vi "Extraction - MainUI.vi"() -> ()   [LabVIEW 2020]
uses:
  File Name Format.ctl
  <vilib>/addons/HF Network Analysis/Support VIs/Read SnP File (SnP).vi
  <vilib>/addons/HF Network Analysis/NI_HFNetworkAnalysis.lvlib
panel:
  in  "Tab Control":enum32{"Main", "Graphs", "Data Table"}(tab)
  in  "Device":T1
  in  "Copy comments":bool caption="Copy comments from \noriginal files (ISD de-embedding)"
  in  "SnP File Path":path
  in  "Filename has to include:":string="_DUT"
  in  "File name format":T2=enum."LV-framework, no file name"
  in  "Model":enum16{"pi", "tee"}(ring)
  in  "Freq for nominal \nvalues (MHz)":dbl=100.0
  in  "Ports":T3(ring)
  in  "Subtract stub":bool
  in  "Inductance (nH)":dbl=0.306
  in  "Capacitance (pF)":dbl=0.04
  out "Horizontal Progress Bar":u8(slide) scale=0.0..100.0
  in  "Play":bool
  in  "Exit":bool
  out "Status":string
  in  "Result File Path":path caption="Result File Path (empty: use the SnP-folder above)"
  in  "File extension":enum16{"Auto", "s1p", "s2p"}(ring)
  in  "Save extraction data":bool=TRUE
  in  "Save file index data":bool=TRUE
  in  "toJMP":bool caption="Save in JMP"
  out "Capa":cluster{"Frequencies (Hz) in":dbl[], dbl[]}[](graph) caption="Capacitance"
  out "R":cluster{"Frequencies (Hz) in":dbl[], dbl[]}(graph) caption="Resistance"
  out "Q":cluster{"Frequencies (Hz) in":dbl[], dbl[]}(graph)
  out "Error Out":errorcluster
  out "Heading":string[](array[string])
  out "Data":string[][](array[string])
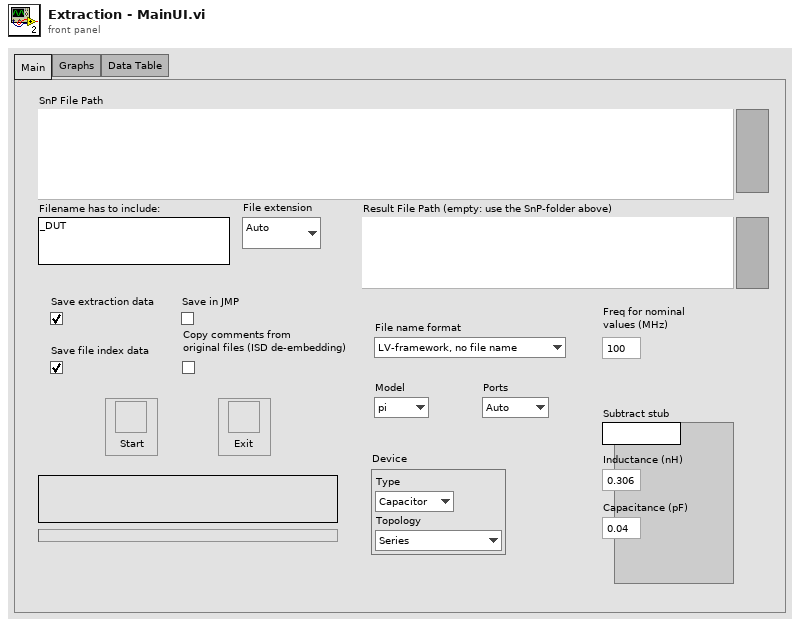
[diagram p1: front panel]
types:
  T1 = cluster{"Type":enum16{"Capacitor", "Switch"}, "Topology":enum16{"Series", "Parallel"}}
  T2 = typedef "File Name Format.ctl" = enum16{"none", "S-para, old", "S-para, new", "S-para, new, step", "ECP", "S-para, new+1", "WS1040", "S-para, new+5100", "S-para, new+5100, no step", "General, space limited", "General, underscore limited", "General, whitespace limited", "LV-framework", "LV-framework, no file name"}
  T3 = enum16{"Auto", "1-Port", "2-Port", "3-port", "4-port"}
  T4 = enum8{"Enabled", "Disabled", "Disabled and Grayed Out"}
  T5 = cluster{cluster{"Frequencies (Hz) in":dbl[], dbl[]}, cluster{"Frequencies (Hz) in":dbl[], dbl[]}, cluster{"Frequencies (Hz) in":dbl[], dbl[]}[]}
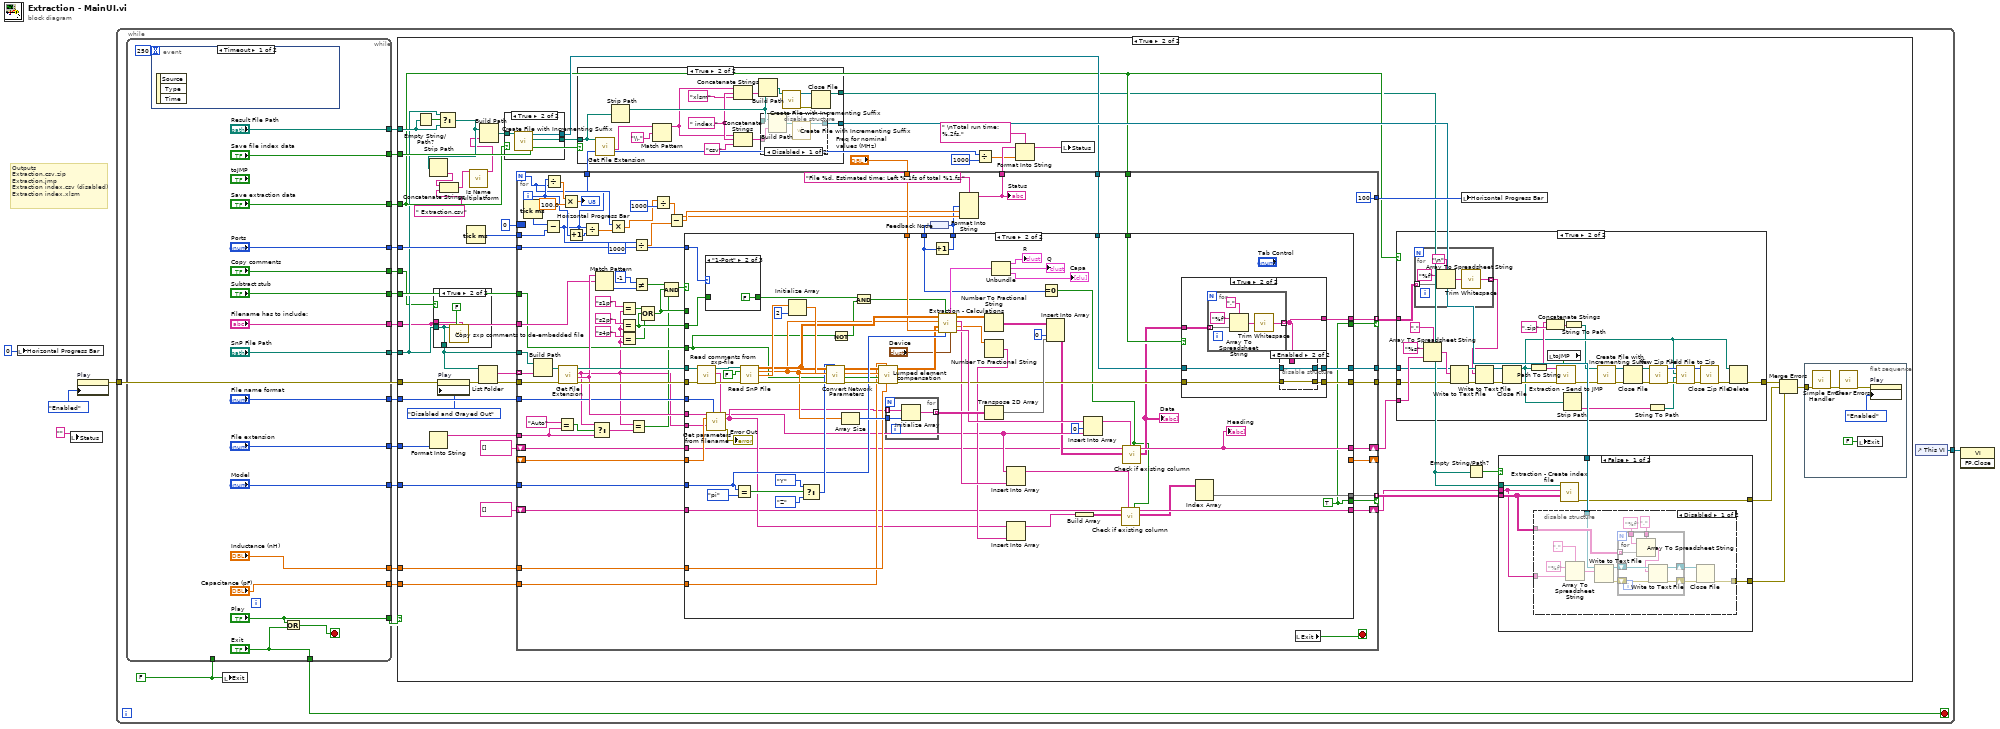
[diagram p0: block diagram]
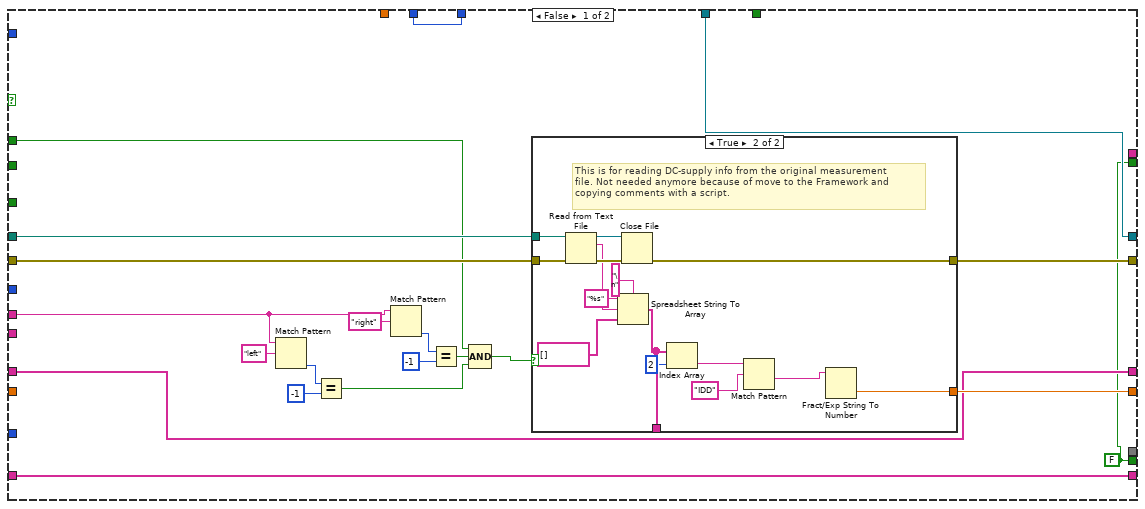
[diagram p10: hidden frame]
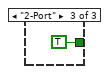
[diagram p13: hidden frame]
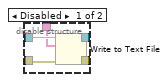
[diagram p15: hidden frame]
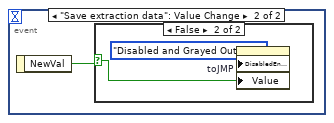
[diagram p16: hidden frame]
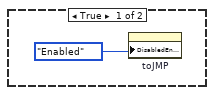
[diagram p17: hidden frame]
diagram:
  # "Outputs\nExtraction.csv.zip\nExtraction.jmp\nExtraction index.csv (disabled)\nExtraction index.xlsm"
  n1 = local write "Horizontal Progress Bar"(u8 0 ("Horizontal Progress Bar")) -> ()
  n2 = local write "Status"("" ("Status")) -> ()
  n3 = property on="Play" class="Bool"("DisabledEnum"=T4."Enabled" ("Disabled")) -> (error out=w3:errorcluster)  [unwired: 2 in, 1 out]
  n4 = while {
    tunnel: w3 -> [w12]
    tunnel: [w10] -> w1
    stop <- w13 stop-if-true
    w11 = FALSE ("Exit")
    n5 = while {
      tunnel: ["SnP File Path"] -> w23
      tunnel: ["Filename has to include:"] -> w22
      tunnel: ["Save extraction data"] -> w21
      tunnel: ["File name format"] -> w20
      tunnel: ["Model"] -> w19
      tunnel: ["Ports"] -> w18
      tunnel: ["Subtract stub"] -> w17
      tunnel: ["Inductance (nH)"] -> w16
      tunnel: ["Capacitance (pF)"] -> w15
      tunnel: ["Play"] -> w14
      tunnel: ["Exit"] -> w13
      tunnel: w11 -> [_]
      tunnel: ["File extension"] -> w9
      tunnel: ["Save file index data"] -> w8
      tunnel: ["Result File Path"] -> w7
      tunnel: ["Copy comments"] -> w6
      stop <- w386 stop-if-true
      n6 = event shown="[0] Timeout" {
        selector: _ -> [_ _]
        dyn-events: _ -> [_ _]
        timeout: 250 -> [_ _]
        event Timeout {
          n7 = event-data() -> ()  [unwired: 1 in, 3 out]
        }
        event "Save extraction data": Value Change {
          n8 = event-data() -> ("NewVal"=w396:bool)  [unwired: 1 in]
          n9 = case shown="False" w396 {
            selector: w396 -> [_ w398]
            frame True {
              n10 = property on="toJMP" class="Bool (strict)"("DisabledEnum"=T4."Enabled" ("Disabled")) -> ()  [unwired: 2 in, 2 out]
            }
            frame False {
              n11 = property on="toJMP" class="Bool (strict)"("DisabledEnum"=T4."Disabled and Grayed Out" ("Disabled"), "Value"=w398) -> ()  [unwired: 2 in, 2 out]
            }
          }
        }
      }
      n12 = Or(x="Play", y="Exit") -> (x .or. y?=w386:bool)
    }
    n13 = local write "Exit"(w11) -> ()
    n14 = case shown="True" w14 {
      tunnel: w23 -> [_ w27]
      tunnel: w22 -> [_ w24]
      tunnel: w21 -> [_ w43]
      tunnel: w20 -> [_ w72]
      tunnel: w19 -> [_ w71]
      tunnel: w18 -> [_ w69]
      tunnel: w17 -> [_ w68]
      tunnel: w16 -> [_ w67]
      tunnel: w15 -> [_ w66]
      tunnel: w12 -> [_ w62]
      tunnel: w9 -> [_ w53]
      tunnel: w8 -> [_ w45]
      tunnel: w7 -> [_ w44]
      tunnel: w6 -> [_ w26]
      frame False {
      }
      frame True {
        n15 = Empty String/Path?(string/path=w44) -> (empty?=w54:bool)
        n16 = Format Into String(w53) -> (resulting string=w52:string)  [unwired: 3 in, 1 out]
        n17 = case shown="True" w26 {
          tunnel: w27 -> [w78 w80]
          tunnel: [w78 w80] -> w25
          tunnel: w24 -> [_ w79]
          frame False {
          }
          frame True {
            n18 = call "Copy sxp comments to de-embedded file.vi"("Filename has to include:"=w79, "Standalone"=FALSE, "SnP File Path"=w80) -> ()  [unwired: 9 in]
          }
        }
        n19 = property on="Play" class="Bool"(error in=w62, "DisabledEnum"=T4."Disabled and Grayed Out" ("Disabled")) -> (error out=w63:errorcluster)  [unwired: 1 in, 1 out]
        n20 = Select(t=w27, s=w54, f=w44) -> (s? t:f=w36:path)
        n21 = Strip Path(path=w36) -> (name=w35:string)  [unwired: 1 out]
        n22 = Concatenate Strings(w35, " Extraction.csv" ("string")) -> (w34:string)
        n23 = Tick Count (ms)() -> (millisecond timer value=w61:u32)
        n24 = call <vilib>:"Is Name Multiplatform.vi"("filename"=w34) -> ("suggested filename"=w32:string)  [unwired: 6 in, 4 out]
        n25 = List Folder(path=w25, error in=w63) -> (filenames=w77:string[], error out=w76:errorcluster)  [unwired: 2 in, 2 out]
        n26 = Build Path(base path=w36, name or relative path=w32) -> (appended path=w75:path)
        n27 = case shown="True" w43 {
          tunnel: w75 -> [w147 w150]
          tunnel: [w147 w149] -> w47
          tunnel: [_ w148] -> w46
          frame False {
          }
          frame True {
            n28 = call <vilib>:"Create File with Incrementing Suffix.vi"("file path"=w150) -> ("actual path"=w149:path, "refnum out"=w148:refnum<file>)  [unwired: 8 in, 1 out]
          }
        }
        n29 = for {
          N -> [w202]
          tunnel: w25 -> [w232]
          tunnel: [w242] -> w73
          tunnel: w76 -> [w237]
          tunnel: w77 -> [w235] mode=indexing
          tunnel: w24 -> [w229]
          shift-right: [w228] -> _
          shift-left: _ -> [w227]
          tunnel: w43 -> [w226]
          tunnel: w46 -> [w225]
          tunnel: [w224] -> w74
          tunnel: w72 -> [w223]
          tunnel: w71 -> [w220]
          tunnel: "Freq for nominal \nvalues (MHz)" -> [w219]
          tunnel: w69 -> [w217]
          tunnel: w68 -> [w216]
          tunnel: w67 -> [w215]
          tunnel: w66 -> [w214]
          tunnel: [u8 100 ("Horizontal Progress Bar")] -> w65
          tunnel: w61 -> [w207]
          tunnel: [w194] -> w59
          tunnel: [w193] -> w58
          tunnel: w52 -> [w190]
          tunnel: [w187] -> w51 mode=indexing if=w186
          border: 0 -> [_]
          shift-right: [w182] -> w31
          shift-left: string[] [] ("Main Heading") -> [w181]
          shift-right: [w185] -> w50
          shift-left: string[] [] ("Main Heading") -> [w180]
          tunnel: [w179] -> w28 mode=indexing if=w178
          i -> [w205]
          stop <- w209 stop-if-true
          n30 = Tick Count (ms)() -> (millisecond timer value=w206:u32)
          n31 = Build Path(base path=w232, name or relative path=w235) -> (appended path=w234:path)
          n32 = Subtract(x=w206, y=w207) -> (x-y=w194:u32)
          n33 = Divide(x=w205, y=w202) -> (x/y=w213:dbl)
          n34 = Equal?(x="Auto" ("y"), y=w190) -> (x = y?=w191:bool)
          n35 = call <vilib>:"Get File Extension.vi"("error in (no error)"=w237, "file"=w234) -> ("error out"=w236:errorcluster, "filename without extension"=w230:string, "lowercase file extension"=w176:string, "dup file"=w231:path)  [unwired: 5 in, 1 out]
          n36 = Multiply(x=w213, y=100.0) -> (x*y=→"Horizontal Progress Bar":dbl)
          n37 = Increment(x=w205) -> (x+1=w204:i32)
          n38 = Divide(x=w194, y=w204) -> (x/y=w203:dbl)
          n39 = Select(t=w176, s=w191, f=w190) -> (s? t:f=w189:string)
          n40 = Match Pattern(string=w230, regular expression=w229) -> (offset past match=w233:i32)  [unwired: 1 in, 3 out]
          n41 = Multiply(x=w202, y=w203) -> (x*y=w196:dbl)
          n42 = Equal?(x="s1p" ("regular expression"), y=w176) -> (x = y?=w221:bool)
          n43 = Equal?(x="s2p" ("regular expression"), y=w176) -> (x = y?=w218:bool)
          n44 = Equal?(x="s4p" ("regular expression"), y=w176) -> (x = y?=w175:bool)
          n45 = Equal?(x=w176, y=w189) -> (x = y?=w188:bool)
          n46 = Divide(x=w194, y=u32 1000) -> (x/y=w199:dbl)
          n47 = Not Equal?(x=-1, y=w233) -> (x != y?=w241:bool)
          n48 = Compound Arithmetic op=OR(w221, w218, w175) -> (w208:bool)
          n49 = Divide(x=w196, y=u32 1000) -> (x/y=w195:dbl)
          n50 = Compound Arithmetic op=AND(w241, w208, w188) -> (w238:bool)
          n51 = Subtract(x=w195, y=w199) -> (x-y=w198:dbl)
          n52 = feedback #1() -> (w184:i32)
          n53 = case shown="True" w238 {
            tunnel: w231 -> [w260 w311]
            tunnel: [w259 w338] -> w242
            tunnel: w236 -> [w261 w312]
            tunnel: w230 -> [w262 w345]
            tunnel: [w258 _] -> w228
            tunnel: w227 -> [_ w339]
            tunnel: w226 -> [_ w337]
            tunnel: w225 -> [w257 w335]
            tunnel: [w257 w334] -> w224
            tunnel: w223 -> [_ w333]
            tunnel: w218 -> [_ w324]
            tunnel: w220 -> [_ w327]
            tunnel: w219 -> [_ w326]
            tunnel: w217 -> [_ w325]
            tunnel: w176 -> [_ w323]
            tunnel: w216 -> [_ w317]
            tunnel: w215 -> [_ w315]
            tunnel: w214 -> [_ w314]
            tunnel: w208 -> [w247 _]
            tunnel: [w244 w291] -> w185
            tunnel: [w243 w283] -> w186
            tunnel: [_ w285] -> w187
            tunnel: w184 -> [w246 w282]
            tunnel: [w246 w307] -> w183
            tunnel: [w245 w296] -> w182
            tunnel: w181 -> [w245 w281]
            tunnel: w180 -> [w244 w289]
            tunnel: [_ w284] -> w179
            tunnel: [w243 w283] -> w178
            frame False {
              w243 = FALSE
              n54 = Match Pattern(string=w262, regular expression="left") -> (offset past match=w254:i32)  [unwired: 1 in, 3 out]
              n55 = Equal?(x=w254, y=-1) -> (x = y?=w249:bool)
              n56 = Match Pattern(string=w262, regular expression="right") -> (offset past match=w251:i32)  [unwired: 1 in, 3 out]
              n57 = Equal?(x=w251, y=-1) -> (x = y?=w250:bool)
              n58 = Compound Arithmetic op=AND(w247, w250, w249) -> (w248:bool)
              n59 = case shown="True" w248 {
                tunnel: w261 -> [w263 w276]
                tunnel: w260 -> [_ w275]
                tunnel: [w263 w274] -> w259
                tunnel: [_ w269] -> _
                tunnel: [_ w264] -> w258
                frame False {
                }
                frame True {
                  # "This is for reading DC-supply info from the original measurement \nfile. Not needed anymore because of move to the Framework and \ncopying comments with a script."
                  n60 = Read from Text File(file (use dialog)=w275, error in=w276) -> (refnum out=w277:refnum<file>, text=w273:string, error out=w278:errorcluster)  [unwired: 2 in, 1 out]
                  n61 = Spreadsheet String To Array(delimiter (Tab)="\n" ("format string"), format string="%s", spreadsheet string=w273, array type (2D Dbl)=string[] []) -> (array=w269:string[])
                  n62 = Close File(refnum=w277, error in=w278) -> (error out=w274:errorcluster)  [unwired: 1 out]
                  n63 = Index Array(array=w269, index=2) -> (element=w266:string)
                  n64 = Match Pattern(string=w266, regular expression="IDD" ("format string")) -> (after substring=w265:string)  [unwired: 1 in, 3 out]
                  n65 = Fract/Exp String To Number(string=w265) -> (number=w264:dbl)  [unwired: 3 in, 1 out]
                }
              }
            }
            frame True {
              w283 = TRUE
              n66 = call "Read comments from sxp-file.vi"("error in (no error)"=w312, "file path"=w311) -> ("error out"=w309:errorcluster, "Comment lines"=w308:string[], "file path out"=w310:path)  [unwired: 7 in]
              n67 = case shown="\"1-Port\"" w325 {
                tunnel: w324 -> [w353 _ _]
                tunnel: [w353 FALSE TRUE] -> w319
                frame "Auto", Default {
                }
                frame "1-Port" {
                }
                frame "2-Port" {
                }
              }
              n68 = call "Get parameters from filename.vi"("Filename"=w345, "File name format"=w333, "Comment lines"=w308, "Idd"=w339, "extension"=w323) -> ("Heading"=w297:string[], "Info"=w298:string[], "Error Out"=→"Error Out":errorcluster)  [unwired: 6 in, 2 out]
              n69 = Equal?(x=w327, y=enum16{"pi", "tee"}."pi") -> (x = y?=w328:bool)
              n70 = call-poly <vilib>:"Read SnP File.vi"("SnP File Path"=w310, "Swap Ports (False)"=FALSE, "Error In"=w309) -> ("S-parameters"=w346:cdb[][], "Frequencies (Hz)"=w322:dbl[], "Z0 (Ohm)"=w350:cdb, "Error Out"=w351:errorcluster)  [unwired: 9 in]
              n71 = Initialize Array(w350, 2 ("dimension size")) -> (w348:cdb[])
              n72 = Select(t=enum16{"Y", "Z"}."Y" ("Parameters to convert"), s=w328, f=enum16{"Y", "Z"}."Z" ("Parameters to convert")) -> (s? t:f=w330:enum16{"Y", "Z"})
              n73 = call "Convert Network Parameters.vi"("Parameters to convert"=w330, "error in (no error)"=w351, "Zc (Ohm)"=w348, "S-par Array In"=w346) -> ("error out"=w336:errorcluster, "Y/Z Array Out"=w320:cdb[][])  [unwired: 5 in, 1 out]
              n74 = Not(x=w317) -> (.not. x?=w316:bool)
              n75 = Array Size(array=w322) -> (size(s)=w344:i32)
              n76 = And(x=w319, y=w316) -> (x .and. y?=w318:bool)
              n77 = call "Lumped element compensation.vi"("Inductance (nH)"=w315, "Capacitance (pF)"=w314, "Subtract stub"=w317, "Frequencies (Hz)"=w322, "Y/Z Array Out in"=w320) -> ("Y/Z Array Out out"=w321:cdb[][])  [unwired: 6 in]
              n78 = for {
                tunnel: w298 -> [w378] mode=indexing
                tunnel: w344 -> [w377]
                tunnel: [w376] -> w342 mode=indexing
                n79 = Initialize Array(w378, w377) -> (w376:string[])
              }
              n80 = Increment(x=w282) -> (x+1=w307:i32)
              n81 = call "Extraction - Calculations.vi"("Device"="Device", "Model"=w327, "2-port?"=w318, "Freq for nominal C (MHz)"=w326, "Y/Z-parameters"=w321, "Frequencies (Hz) in"=w322, "S-parameters"=w346) -> ("Heading"=w340:string[], "index file values"=w300:dbl[], "index file heading"=w301:string[], "Frequency,C, R, Q/-IL, L, Cshunt1/2, Rshunt1/2, Lshunt1/2, SRF"=w306:dbl[][], "Graphs"=w305:T5)
              n82 = Number To Fractional String(number=w306) -> (F-format string=w347:string[][])  [unwired: 3 in]
              n83 = Number To Fractional String(number=w300) -> (F-format string=w299:string[])  [unwired: 3 in]
              n84 = Transpose 2D Array(2D array=w342) -> (transposed array=w343:string[][])
              n85 = Unbundle(w305) -> (→"R":cluster{"Frequencies (Hz) in":dbl[], dbl[]}, →"Q":cluster{"Frequencies (Hz) in":dbl[], dbl[]}, →"Capa":cluster{"Frequencies (Hz) in":dbl[], dbl[]}[])
              n86 = Insert Into Array(array=w297, new element=w301) -> (w290:string[])  [unwired: 1 in]
              n87 = Insert Into Array(array=w298, new element=w299) -> (w288:string[])  [unwired: 1 in]
              n88 = Equal To 0?(x=w282) -> (x = 0?=w280:bool)
              n89 = Insert Into Array(array=w347, index (col)=0 ("disabled index (col)"), new element=w343) -> (w293:string[][])  [unwired: 1 in]
              n90 = Build Array(w288) -> (w287:string[][])
              n91 = Insert Into Array(array=w340, index=0, new element=w297) -> (w294:string[])
              n92 = call "Check if existing column.vi"("Init"=w280, "New Heading"=w290, "New Data"=w287, "Main Heading in"=w289) -> ("New Data out"=w286:string[][], "Main Heading"=w291:string[])  [unwired: 6 in]
              n93 = call "Check if existing column.vi"("Init"=w280, "New Heading"=w294, "New Data"=w293, "Main Heading in"=w281) -> ("New Data out"=w292:string[][], "Main Heading"=w296:string[])  [unwired: 6 in]
              "Data" <- w292
              "Heading" <- w296
              n94 = case shown="True" w337 {
                tunnel: [w357 w360] -> w338
                tunnel: w292 -> [_ w363]
                tunnel: w336 -> [w357 w362]
                tunnel: w335 -> [w356 w361]
                tunnel: [w356 w359] -> w334
                tunnel: [_ w358] -> w284
                frame False {
                }
                frame True {
                  n95 = for {
                    tunnel: w363 -> [w373] mode=indexing
                    tunnel: [w371] -> w358 mode=indexing
                    n96 = Array To Spreadsheet String(delimiter (Tab)=",", array=w373, 3:"%f" ("format string")) -> (spreadsheet string=w372:string)
                    n97 = call <vilib>:"Trim Whitespace.vi"("string"=w372) -> ("trimmed string"=w371:string)  [unwired: 1 in]
                  }
                  n98 = disable-structure shown="Enabled" {
                    disable-tunnel: w362 -> [w368 w369]
                    disable-tunnel: w361 -> [w367 w370]
                    disable-tunnel: [w366 w369] -> w360
                    disable-tunnel: [w365 w370] -> w359
                    disable-tunnel: w358 -> [w364 _]
                    frame Disabled {
                      n99 = Write to Text File(file (use dialog)=w367, text=w364, error in=w368) -> (refnum out=w365:refnum<file>, error out=w366:errorcluster)  [unwired: 1 in, 1 out]
                    }
                    frame Enabled {
                    }
                  }
                }
              }
              n100 = Index Array(array=w286) -> (element=w285:string[])  [unwired: 2 in]
            }
          }
          n101 = feedback-in #1(w183) -> ()
          n102 = Format Into String(format string="File %d. Estimated time: Left %.1fs of total %1.fs.", w183, w198, w195) -> (resulting string=w193:string)  [unwired: 2 in, 1 out]
          "Status" <- w193
          n103 = local read "Exit"() -> (w209:bool)
        }
        n104 = case shown="True" w45 {
          tunnel: [_ w169] -> w49
          tunnel: [_ w161] -> w38
          tunnel: w47 -> [_ w160]
          frame False {
          }
          frame True {
            w165 = " index." ("string")
            n105 = call <vilib>:"Get File Extension.vi"("file"=w160) -> ("filename without extension"=w158:string)  [unwired: 6 in, 4 out]
            n106 = Strip Path(path=w160) -> (stripped path=w166:path)  [unwired: 1 out]
            n107 = Match Pattern(string=w158, regular expression="\\.") -> (before substring=w157:string)  [unwired: 1 in, 3 out]
            n108 = Concatenate Strings(w157, w165, "xlsm" ("string")) -> (w167:string)
            n109 = Concatenate Strings(w157, w165, "csv" ("string")) -> (w170:string)
            n110 = Build Path(base path=w166, name or relative path=w167) -> (appended path=w168:path)
            n111 = disable-structure shown="Disabled" {
              disable-tunnel: w170 -> [w173 _]
              disable-tunnel: [w172 _] -> w169
              disable-tunnel: w166 -> [w171 _]
              frame Disabled {
                n112 = Build Path(base path=w171, name or relative path=w173) -> (appended path=w174:path)
                n113 = call <vilib>:"Create File with Incrementing Suffix.vi"("file path"=w174) -> ("refnum out"=w172:refnum<file>)  [unwired: 8 in, 2 out]
              }
              frame Enabled {
              }
            }
            n114 = call <vilib>:"Create File with Incrementing Suffix.vi"("file path"=w168) -> ("error out"=w162:errorcluster, "refnum out"=w163:refnum<file>)  [unwired: 8 in, 1 out]
            n115 = Close File(refnum=w163, error in=w162) -> (path=w161:path)  [unwired: 1 out]
          }
        }
        n116 = Divide(x=w59, y=u32 1000) -> (x/y=w55:dbl)
        n117 = Format Into String(format string=" \nTotal run time: %.2fs.", initial string=w58, w55) -> (resulting string=w57:string)  [unwired: 1 in, 1 out]
        n118 = local write "Status"(w57) -> ()
        n119 = case shown="True" w43 {
          tunnel: w74 -> [_ w135]
          tunnel: w73 -> [w109 w134]
          tunnel: [w109 w117] -> w40
          tunnel: w31 -> [_ w137]
          tunnel: w28 -> [_ w129]
          frame False {
          }
          frame True {
            n120 = for {
              tunnel: w129 -> [w144] mode=indexing
              tunnel: [w142] -> w128 mode=indexing
              n121 = Array To Spreadsheet String(delimiter (Tab)="\n", array=w144, 3:"%f" ("format string")) -> (spreadsheet string=w143:string)
              n122 = call <vilib>:"Trim Whitespace.vi"("string"=w143) -> ("trimmed string"=w142:string)  [unwired: 1 in]
            }
            n123 = Array To Spreadsheet String(delimiter (Tab)=",", array=w137, 3:"%s" ("format string")) -> (spreadsheet string=w136:string)
            n124 = Write to Text File(file (use dialog)=w135, text=w136, error in=w134) -> (refnum out=w133:refnum<file>, error out=w132:errorcluster)  [unwired: 1 in, 1 out]
            n125 = Write to Text File(file (use dialog)=w133, text=w128, error in=w132) -> (refnum out=w131:refnum<file>, error out=w130:errorcluster)  [unwired: 1 in, 1 out]
            n126 = Close File(refnum=w131, error in=w130) -> (path=w116:path, error out=w140:errorcluster)
            n127 = Path To String(path=w116) -> (string=w119:string)
            n128 = Concatenate Strings(w119, ".zip" ("name or relative path")) -> (w126:string)
            n129 = local read "toJMP"() -> (w141:bool)
            n130 = call "Extraction - Send to JMP.vi"("Send to JMP"=w141, "Error In"=w140, "filename"=w119) -> ("Error Out"=w111:errorcluster)  [unwired: 8 in]
            n131 = Strip Path(path=w116) -> (name=w121:string)  [unwired: 1 out]
            n132 = String To Path(string=w126) -> (path=w113:path)
            n133 = call <vilib>:"Create File with Incrementing Suffix.vi"("error in (no error)"=w111, "file path"=w113) -> ("error out"=w114:errorcluster, "refnum out"=w115:refnum<file>)  [unwired: 7 in, 1 out]
            n134 = Close File(refnum=w115, error in=w114) -> (path=w112:path, error out=w110:errorcluster)
            n135 = String To Path(string=w121) -> (path=w120:path)
            n136 = call <vilib>:"New Zip File.vi"("error in (no error)"=w110, "target"=w112) -> ("error out"=w125:errorcluster, "zip file out"=w124:i64)  [unwired: 3 in, 1 out]
            n137 = call <vilib>:"Add File to Zip.vi"("error in (no error)"=w125, "destination path in zip"=w120, "source file path"=w116, "zip file in"=w124) -> ("error out"=w122:errorcluster, "zip file out"=w123:i64)  [unwired: 6 in]
            n138 = call <vilib>:"Close Zip File.vi"("error in (no error)"=w122, "zip file in"=w123) -> ("error out"=w118:errorcluster)  [unwired: 5 in]
            n139 = Delete(path (use dialog)=w116, error in=w118) -> (error out=w117:errorcluster)  [unwired: 3 in, 2 out]
          }
        }
        n140 = local write "Horizontal Progress Bar"(w65) -> ()
        n141 = Empty String/Path?(string/path=w38) -> (empty?=w37:bool)
        n142 = case shown="False" w37 {
          tunnel: w51 -> [w87 _]
          tunnel: w38 -> [w86 _]
          tunnel: w50 -> [w85 _]
          tunnel: w49 -> [w84 _]
          tunnel: [w83 _] -> w42
          tunnel: [w82 _] -> w41
          frame False {
            n143 = disable-structure shown="Disabled" {
              disable-tunnel: w87 -> [w100 _]
              disable-tunnel: w85 -> [w99 _]
              disable-tunnel: w84 -> [w98 _]
              disable-tunnel: [w88 _] -> w83
              frame Disabled {
                n144 = Array To Spreadsheet String(delimiter (Tab)=",", array=w99, 3:"%f" ("format string")) -> (spreadsheet string=w91:string)
                n145 = Write to Text File(file (use dialog)=w98, text=w91) -> (refnum out=w96:refnum<file>, error out=w97:errorcluster)  [unwired: 2 in, 1 out]
                n146 = for {
                  tunnel: w100 -> [w102] mode=indexing
                  shift-right: [w106] -> w95
                  shift-left: w96 -> [w107]
                  shift-right: [w105] -> w94
                  shift-left: w97 -> [w108]
                  tunnel: "," ("delimiter (Tab)") -> [w104]
                  tunnel: "%f" ("format string") -> [w103]
                  n147 = Array To Spreadsheet String(delimiter (Tab)=w104, array=w102, 3:w103) -> (spreadsheet string=w101:string)
                  n148 = Write to Text File(file (use dialog)=w107, text=w101, error in=w108) -> (refnum out=w106:refnum<file>, error out=w105:errorcluster)  [unwired: 1 in, 1 out]
                }
                n149 = Close File(refnum=w95, error in=w94) -> (error out=w88:errorcluster)  [unwired: 1 out]
              }
              frame Enabled {
              }
            }
            n150 = call "Extraction - Create index file.vi"("Data"=w87, "Heading"=w85, "report file path"=w86) -> ("Error Out"=w82:errorcluster)  [unwired: 8 in]
          }
          frame True {
          }
        }
        n151 = Merge Errors(w40, w41, w42) -> (w39:errorcluster)
        n152 = flat-sequence {
          tunnel: w39 -> [w152]
          frame #0 {
            n153 = call <vilib>:"Simple Error Handler.vi"("error in (no error)"=w152) -> ("error out"=w154:errorcluster)  [unwired: 4 in, 4 out]
            n154 = call <vilib>:"Clear Errors.vi"("error in (no error)"=w154) -> ("error out"=w153:errorcluster)  [unwired: 5 in, 1 out]
            n155 = local write "Exit"(FALSE ("Exit")) -> ()
            n156 = property on="Play" class="Bool"(error in=w153, "DisabledEnum"=T4."Enabled" ("Disabled")) -> ()  [unwired: 1 in, 2 out]
          }
        }
      }
    }
    n157 = control-ref of="This VI"() -> (w10:refnum<vi>)
  }
  n158 = invoke class="VI" method="FP.Close"(reference=w1) -> ()  [unwired: 2 in, 3 out]
